vi "Create.vi"(8 "error in (no error)":errorcluster) -> (0 "error out":errorcluster, 3 "Messenger out":refnum<class "Messenger.lvclass">)   [LabVIEW 2015, in "Messenger.lvclass"]
uses:
  Messenger.lvclass
  Message/Message.lvclass
  Messenger.lvclass/Messenger.ctl
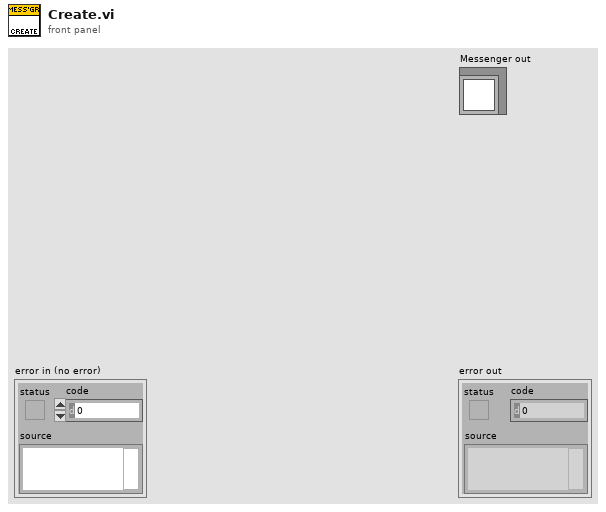
[diagram p1: front panel]
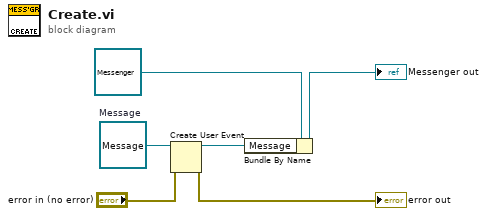
[diagram p0: block diagram]
diagram:
  w2 = refnum<class "Message.lvclass"> refnum  # Message
  n1 = Create User Event(user event datatype=w2, error in="error in (no error)") -> (user event=w1:refnum<user-event>, error out=→"error out":errorcluster)
  n2 = Bundle By Name(cluster=refnum<class "Messenger.lvclass"> refnum ("Messenger in"), "Message"=w1) -> (→"Messenger out":refnum<class "Messenger.lvclass">)
